vi "escapi_open_camera.vi"(8 "error in (no error)":errorcluster, 10 "Config path":path, 11 "camera_name":string) -> (0 "error out":errorcluster, 2 "height":i32, 3 "width":i32)   [LabVIEW 2022 SP3, in "Vision.lvlib"]
uses:
  Vision.lvlib
  <vilib>/Utility/config.llb/Read Key (String).vi
  <vilib>/Utility/config.llb/Read Key (I32).vi
  bin/Vision.dll
  <vilib>/Utility/config.llb/NI_LVConfig.lvlib
panel:
  out "file created?":bool
  out "found?":bool
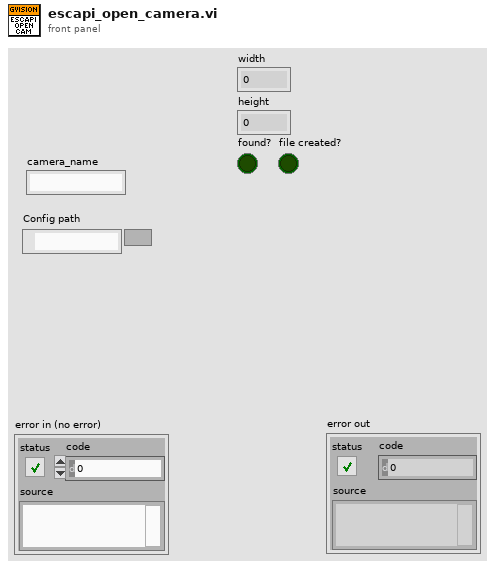
[diagram p1: front panel]
types:
  T1 = typedef "NI_LVConfig.lvlib/Config Data RefNum.ctl" = refnum<k1>
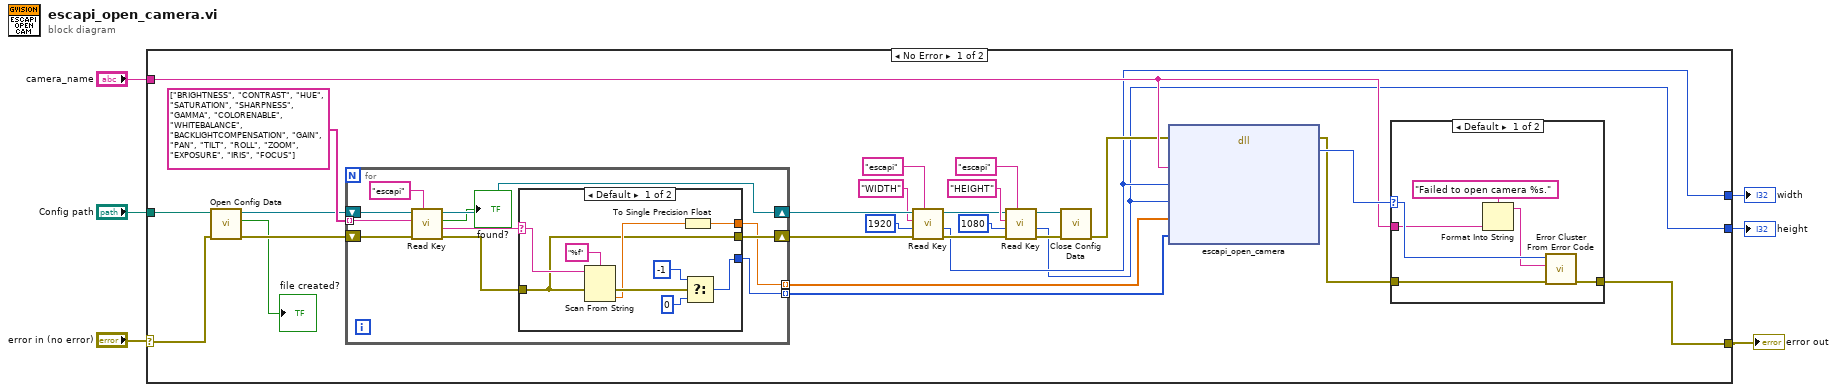
[diagram p0: block diagram]
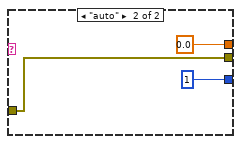
[diagram p2: hidden frame]
diagram:
  n1 = case shown="No Error" "error in (no error)" {
    selector: "error in (no error)" -> [w29 w64]
    tunnel: [w31 w64] -> w4
    tunnel: "camera_name" -> [w24 _]
    tunnel: "Config path" -> [w30 _]
    tunnel: [w9 _] -> w2
    tunnel: [w8 _] -> w1
    frame No Error {
      n2 = call <vilib>:"Open Config Data.vi"("error in (no error)"=w29, "configuration file path"=w30) -> ("error out"=w26:errorcluster, "file created?"=→"file created?":bool, "refnum"=w27:T1)  [unwired: 7 in]
      n3 = for {
        tunnel: string[] ["BRIGHTNESS", "CONTRAST", "HUE", "SATURATION", "SHARPNESS", "GAMMA", "COLORENABLE", "WHITEBALANCE", "BACKLIGHTCOMPENSATION", "GAIN", "PAN", "TILT", "ROLL", "ZOOM", "EXPOSURE", "IRIS", "FOCUS"] -> [w43] mode=indexing
        shift-right: [w39] -> w22
        shift-left: w27 -> [w44]
        shift-right: [w37] -> w21
        shift-left: w26 -> [w41]
        tunnel: [w36] -> w25 mode=indexing
        tunnel: [w35] -> w23 mode=indexing
        n4 = call-poly <vilib>:"Read Key.vi"("section"="escapi", "error in (no error)"=w41, "key"=w43, "refnum"=w44) -> ("error out"=w38:errorcluster, "value"=w40:string, "found?"=→"found?":bool, "refnum out"=w39:T1)  [unwired: 4 in]
        n5 = case shown="Default" w40 {
          selector: w40 -> [w53 _]
          tunnel: [w46 1] -> w35
          tunnel: [w51 sgl 0.0] -> w36
          tunnel: w38 -> [w45 w54]
          tunnel: [w45 w54] -> w37
          frame Default {
            n6 = Scan From String(format string="%f", input string=w53, error in=w45) -> (error out=w50:errorcluster, output 1=w49:dbl)  [unwired: 2 in, 2 out]
            n7 = To Single Precision Float(number=w49) -> (single precision float=w51:sgl)
            n8 = Select(t=-1, s=w50, f=0) -> (s? t:f=w46:i32)
          }
          frame "auto" {
          }
        }
      }
      n9 = call-poly <vilib>:"Read Key.vi"("section"="escapi", "error in (no error)"=w21, "default value"=1920, "key"="WIDTH", "refnum"=w22) -> ("error out"=w13:errorcluster, "value"=w9:i32, "refnum out"=w14:T1)  [unwired: 3 in, 1 out]
      n10 = call-poly <vilib>:"Read Key.vi"("section"="escapi", "error in (no error)"=w13, "default value"=1080, "key"="HEIGHT", "refnum"=w14) -> ("error out"=w11:errorcluster, "value"=w8:i32, "refnum out"=w12:T1)  [unwired: 3 in, 1 out]
      n11 = call <vilib>:"Close Config Data.vi"("error in (no error)"=w11, "refnum"=w12) -> ("error out"=w10:errorcluster)  [unwired: 8 in, 1 out]
      n12 = dll-call lib="C:/Users/Caleb/Desktop/nebraska-silicon-lab/pixel-gantry-extra/LV/bin/Vision.dll" fn="escapi_open_camera"(error in=w10, "camera_name"=w24, "width"=w9, "height"=w8, "props"=w25, "prop_autos"=w23) -> (error out=w32:errorcluster, "return type"=w33:i32)  [unwired: 7 in, 1 out]
      n13 = case shown="Default" w33 {
        selector: w33 -> [w60 _]
        tunnel: w32 -> [w62 w63]
        tunnel: [w61 w63] -> w31
        tunnel: w24 -> [w58 _]
        frame Default {
          n14 = Format Into String(format string="Failed to open camera %s." ("error message (\"\")"), w58) -> (resulting string=w57:string)  [unwired: 2 in, 1 out]
          n15 = call <vilib>:"Error Cluster From Error Code.vi"("error in (no error)"=w62, "error message (\"\")"=w57, "error code (0)"=w60) -> ("error out"=w61:errorcluster)  [unwired: 6 in]
        }
        frame 0 {
        }
      }
    }
    frame Error {
    }
  }
  "error out" <- w4
  "width" <- w2
  "height" <- w1
